vi "XBEE Tx Serial Frame Processor.vi"(9 "TX Frame Queue":refnum<queue>, 11 "VISA Serial Port":refnum<visa-resource-name>) -> (0 "error out":errorcluster)   [LabVIEW 2021]
uses:
  WiFi API Frame.ctl
  WiFi API Frame Type.ctl
  stop button.vi
panel:
  in  "stop":bool
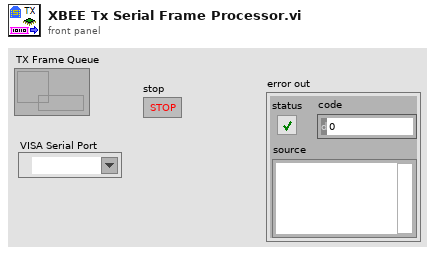
[diagram p1: front panel]
types:
  T1 = typedef "WiFi API Frame.ctl" = cluster{"Length":u16, "Frame Type":T2, "Payload":u8[], "Checksum":u8}
  T2 = typedef "WiFi API Frame Type.ctl" = u8
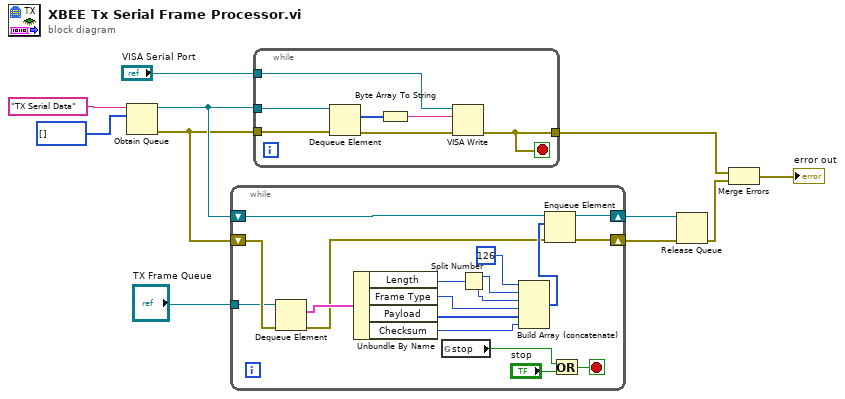
[diagram p0: block diagram]
diagram:
  n1 = Obtain Queue(name (unnamed)="TX Serial Data", element data type=u8[] []) -> (queue out=w9:refnum<queue>, error out=w6:errorcluster)  [unwired: 3 in, 1 out]
  n2 = while {
    shift-right: [w27] -> w8
    shift-left: w9 -> [w29]
    shift-right: [w26] -> w7
    shift-left: w6 -> [w28]
    tunnel: "TX Frame Queue" -> [w16]
    stop <- w13 stop-if-true
    n3 = Dequeue Element(queue=w16, error in (no error)=w28) -> (element=w15:T1, error out=w14:errorcluster)  [unwired: 1 in, 2 out]
    n4 = Unbundle By Name(w15) -> ("Length"=w25:u16, "Frame Type"=w22:T2, "Payload"=w21:u8[], "Checksum"=w20:u8)
    n5 = global read "stop button.vi" "stop"() -> (w12:bool)
    n6 = Split Number(x=w25) -> (hi(x)=w24:u8, lo(x)=w23:u8)
    n7 = Build Array (concatenate)(u8 126, w24, w23, w22, w21, w20) -> (w19:T2[])
    n8 = Enqueue Element(queue=w29, element=w19, error in (no error)=w14) -> (queue out=w27:refnum<queue>, error out=w26:errorcluster)  [unwired: 1 in, 1 out]
    n9 = Or(x=w12, y="stop") -> (x .or. y?=w13:bool)
  }
  n10 = while {
    tunnel: "VISA Serial Port" -> [w35]
    tunnel: w9 -> [w36]
    tunnel: w6 -> [w34]
    tunnel: [w32] -> w1
    stop <- w32 stop-if-true
    n11 = Dequeue Element(queue=w36, error in (no error)=w34) -> (element=w33:u8[], error out=w30:errorcluster)  [unwired: 1 in, 2 out]
    n12 = Byte Array To String(unsigned byte array=w33) -> (string=w31:string)
    n13 = VISA Write(VISA resource name=w35, write buffer=w31, error in (no error)=w30) -> (error out=w32:errorcluster)  [unwired: 2 out]
  }
  n14 = Release Queue(queue=w8, error in (no error)=w7) -> (error out=w2:errorcluster)  [unwired: 1 in, 2 out]
  n15 = Merge Errors(w1, w2) -> (→"error out":errorcluster)
